vi "ep_Public Record Inf to String.vi"(8 "error in":errorcluster, 11 "task in":T1={"file refnums"=[], "Data Object"=refnum, "config info"={"station_name"="", "rec_dev_id"="", "rev_year"=1999.0, "TT"=0, "##A"=0, "##D"=0, "analog channel info"=[], "status channel info"=[], "lf"=-inf, "nrates"=65535, "samp info"=[], "initial timestamp"=timestamp(0 s since 1904-01-01), "trigger timestamp"=timestamp(0 s since 1904-01-01), "ft"=enum."Binary", "timemult"=1.0}, "public inf content"={"Source"="", "Record Type"=enum."Fault", "Phase ID"="", "Event Description"="", "Device ID"="", "Distance of Fault"=-1.0, "Distance Unit"=enum."Miles", "Max_Current"=inf, "Min_Current"=-inf, "Max_Voltage"=inf, "Min_Voltage"=-inf, "EventNoteCount"=0, "Event Information"=[]}, "private inf content"=[], "internal buffers"={"start index"=1, "config to public inf"=enum."disabled", "static config info"="", "static file_des record inf"="", "static file_des channel inf"="", "public inf"="", "private inf"=""}} {"public inf content"."Event Information"."min sample number" max=9999999999; "public inf content"."Event Information"."max sample number" max=9999999999; "config info"."nrates" max=999; "config info"."status channel info"."Dn" min=1 max=999999; "config info"."analog channel info"."An" min=1 max=999999; "config info"."trigger timestamp" format="%<%H:%M:%S%6u\n%d/%m/%Y>T"; "config info"."initial timestamp" format="%<%H:%M:%S%6u\n%d/%m/%Y>T"; "config info"."##D" max=999999; "config info"."##A" max=999999; "config info"."TT" min=1 max=999999; "config info"."rev_year" min=1999.0 max=1999.0}) -> (0 "error out":errorcluster, 2 "public record inf":string, 3 "dup task":T1={"file refnums"=[], "Data Object"=refnum, "config info"={"station_name"="", "rec_dev_id"="", "rev_year"=1999.0, "TT"=0, "##A"=0, "##D"=0, "analog channel info"=[], "status channel info"=[], "lf"=-inf, "nrates"=65535, "samp info"=[], "initial timestamp"=timestamp(0 s since 1904-01-01), "trigger timestamp"=timestamp(0 s since 1904-01-01), "ft"=enum."Binary", "timemult"=1.0}, "public inf content"={"Source"="", "Record Type"=enum."Fault", "Phase ID"="", "Event Description"="", "Device ID"="", "Distance of Fault"=-1.0, "Distance Unit"=enum."Miles", "Max_Current"=inf, "Min_Current"=-inf, "Max_Voltage"=inf, "Min_Voltage"=-inf, "EventNoteCount"=0, "Event Information"=[]}, "private inf content"=[], "internal buffers"={"start index"=1, "config to public inf"=enum."disabled", "static config info"="", "static file_des record inf"="", "static file_des channel inf"="", "public inf"="", "private inf"=""}} {"public inf content"."Event Information"."min sample number" max=9999999999; "public inf content"."Event Information"."max sample number" max=9999999999; "config info"."nrates" max=999; "config info"."status channel info"."Dn" min=1 max=999999; "config info"."analog channel info"."An" min=1 max=999999; "config info"."trigger timestamp" format="%<%H:%M:%S%6u\n%d/%m/%Y>T"; "config info"."initial timestamp" format="%<%H:%M:%S%6u\n%d/%m/%Y>T"; "config info"."##D" max=999999; "config info"."##A" max=999999; "config info"."TT" min=1 max=999999; "config info"."rev_year" min=1999.0 max=1999.0})   [LabVIEW 2014, in "NI_EP_COMTRADE.lvlib"]
uses:
  <vilib>/addons/Electrical Power/File IO/NI_EP_COMTRADE.lvlib
  <vilib>/addons/Electrical Power/File IO/COMTRADE/typedefs/ep_Task.ctl
  <vilib>/addons/Electrical Power/File IO/COMTRADE/typedefs/ep_Config Info.ctl
  <vilib>/addons/Electrical Power/File IO/COMTRADE/typedefs/ep_Analog Channel Info.ctl
  <vilib>/addons/Electrical Power/File IO/COMTRADE/typedefs/ep_Status Channel Info.ctl
  <vilib>/addons/Electrical Power/File IO/COMTRADE/typedefs/ep_File Format.ctl
  <vilib>/addons/Electrical Power/File IO/COMTRADE/typedefs/ep_Public Inf Content.ctl
  <vilib>/addons/Electrical Power/File IO/COMTRADE/typedefs/ep_Public Event Inf.ctl
  <vilib>/addons/Electrical Power/File IO/COMTRADE/typedefs/ep_Private Inf Content.ctl
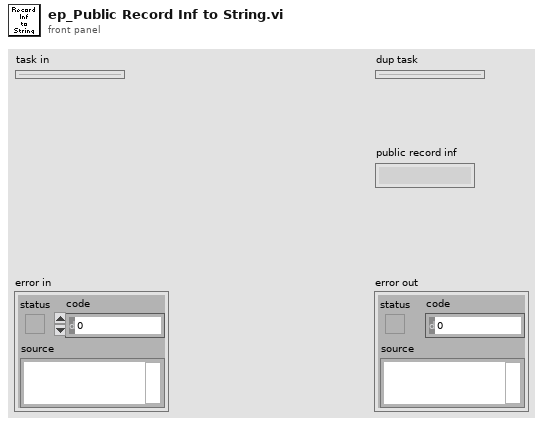
[diagram p1: front panel]
types:
  T1 = typedef "NI_EP_COMTRADE.lvlib/ep_Task.ctl" = cluster{"file refnums":refnum<file>[], "Data Object":refnum<k20>, "config info":T2, "public inf content":T6, "private inf content":T8, "internal buffers":cluster{"start index":u32, "config to public inf":enum16{"disabled", "enabled", "buffered"}, "static config info":string, "static file_des record inf":string, "static file_des channel inf":string, "public inf":string, "private inf":string}}
  T2 = typedef "NI_EP_COMTRADE.lvlib/ep_Config Info.ctl" = cluster{"station_name":string, "rec_dev_id":string, "rev_year":dbl, "TT":u32, "##A":u32, "##D":u32, "analog channel info":T3[], "status channel info":T4[], "lf":sgl, "nrates":u16, "samp info":cluster{"samp":sgl, "endsamp":u32}[], "initial timestamp":timestamp, "trigger timestamp":timestamp, "ft":T5, "timemult":sgl}
  T3 = typedef "NI_EP_COMTRADE.lvlib/ep_Analog Channel Info.ctl" = cluster{"An":u32, "ch_id":string, "ph":string, "ccbm":string, "uu":string, "a":sgl, "b":sgl, "skew":sgl, "min":i32, "max":i32, "primary":sgl, "secondary":sgl, "PS":enum16{"P", "S"}}
  T4 = typedef "NI_EP_COMTRADE.lvlib/ep_Status Channel Info.ctl" = cluster{"Dn":u32, "ch_id":string, "ph":string, "ccbm":string, "Y":bool}
  T5 = typedef "NI_EP_COMTRADE.lvlib/ep_File Format.ctl" = enum16{"ASCII", "Binary"}
  T6 = typedef "NI_EP_COMTRADE.lvlib/ep_Public Inf Content.ctl" = cluster{"Source":string, "Record Type":enum16{"Fault", "Unknown", "Misoperation", "Close", "Trip", "Reclose", "Power swing", "Simulation"}, "Phase ID":string, "Event Description":string, "Device ID":string, "Distance of Fault":dbl, "Distance Unit":enum16{"Miles", "Kilometers", "Percent of line", "Percent of setting", "Ohms"}, "Max_Current":dbl, "Min_Current":dbl, "Max_Voltage":dbl, "Min_Voltage":dbl, "EventNoteCount":u32, "Event Information":T7[]}
  T7 = typedef "NI_EP_COMTRADE.lvlib/ep_Public Event Inf.ctl" = cluster{"channel number":u32, "max value":dbl, "min value":dbl, "max sample number":u64, "min sample number":u64, "max sample text":string[], "min sample text":string[]}
  T8 = typedef "NI_EP_COMTRADE.lvlib/ep_Private Inf Content.ctl" = cluster{"Section Header":string, "Entry Names":string[], "Entry Values":string[]}[]
  T9 = enum16{"Fault", "Unknown", "Misoperation", "Close", "Trip", "Reclose", "Power Swing", "Simulation"}
  T10 = enum16{"Fault", "Unknown", "Misoperation", "Close", "Trip", "Reclose", "Power swing", "Simulation"}
  T11 = enum16{"Miles", "Kilometers", "Percent of line", "Percent of setting", "Ohms"}
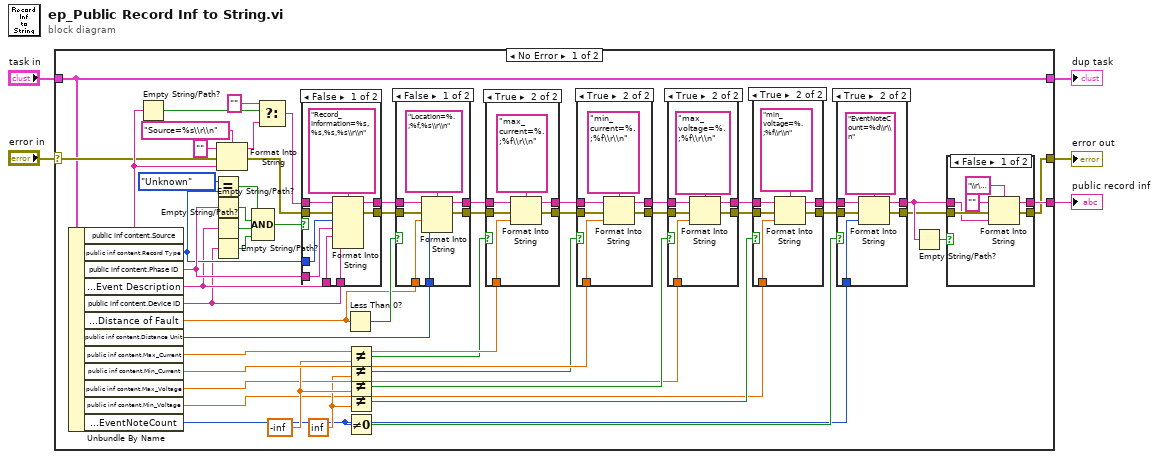
[diagram p0: block diagram]
diagram:
  n1 = case shown="No Error" "error in" {
    selector: "error in" -> [w38 w126]
    tunnel: "task in" -> [w37 w127]
    tunnel: [w37 w127] -> w3
    tunnel: [w6 w126] -> w2
    tunnel: [w9 _] -> w1
    frame No Error {
      w19 = inf ("y")
      w24 = -inf ("y")
      n2 = Unbundle By Name(w37) -> ("public inf content.Source"=w47:string, "public inf content.Record Type"=w43:T10, "public inf content.Phase ID"=w52:string, "public inf content.Event Description"=w36:string, "public inf content.Device ID"=w35:string, "public inf content.Distance of Fault"=w33:dbl, "public inf content.Distance Unit"=w34:T11, "public inf content.Max_Current"=w30:dbl, "public inf content.Min_Current"=w26:dbl, "public inf content.Max_Voltage"=w20:dbl, "public inf content.Min_Voltage"=w15:dbl, "public inf content.EventNoteCount"=w12:u32)
      n3 = Empty String/Path?(string/path=w47) -> (empty?=w49:bool)
      n4 = Equal?(x=T9."Unknown" ("y"), y=w43) -> (x = y?=w56:bool)
      n5 = Empty String/Path?(string/path=w52) -> (empty?=w55:bool)
      n6 = Empty String/Path?(string/path=w36) -> (empty?=w54:bool)
      n7 = Empty String/Path?(string/path=w35) -> (empty?=w46:bool)
      n8 = Format Into String(format string="Source=%s\\r\\n", initial string="", error in=w38, w47) -> (resulting string=w50:string, error out=w44:errorcluster)
      n9 = Compound Arithmetic op=AND(w56, w55, w54, w46) -> (w53:bool)
      n10 = Select(t="", s=w49, f=w50) -> (s? t:f=w45:string)
      n11 = case shown="False" w53 {
        tunnel: w43 -> [w123 _]
        tunnel: w52 -> [w119 _]
        tunnel: w45 -> [w121 w125]
        tunnel: w44 -> [w120 w124]
        tunnel: [w118 w124] -> w40
        tunnel: [w117 w125] -> w39
        tunnel: w36 -> [w116 _]
        tunnel: w35 -> [w115 _]
        frame False {
          n12 = Format Into String(format string="Record_Information=%s,%s,%s,%s\\r\\n", initial string=w121, error in=w120, w123, w119, w116, w115) -> (resulting string=w117:string, error out=w118:errorcluster)
        }
        frame True {
        }
      }
      n13 = Less Than 0?(x=w33) -> (x < 0?=w41:bool)
      n14 = Not Equal?(x=w30, y=w24) -> (x != y?=w27:bool)
      n15 = Not Equal?(x=w26, y=w19) -> (x != y?=w25:bool)
      n16 = Not Equal?(x=w20, y=w24) -> (x != y?=w21:bool)
      n17 = Not Equal?(x=w15, y=w19) -> (x != y?=w16:bool)
      n18 = Not Equal To 0?(x=w12) -> (x != 0?=w13:bool)
      n19 = case shown="False" w41 {
        tunnel: [w112 w114] -> w31
        tunnel: w40 -> [w109 w114]
        tunnel: [w110 w113] -> w32
        tunnel: w39 -> [w111 w113]
        tunnel: w34 -> [w108 _]
        tunnel: w33 -> [w107 _]
        frame False {
          n20 = Format Into String(format string="Location=%.;%f,%s\\r\\n", initial string=w111, error in=w109, w107, w108) -> (resulting string=w110:string, error out=w112:errorcluster)
        }
        frame True {
        }
      }
      n21 = case shown="True" w27 {
        tunnel: [w99 w105] -> w28
        tunnel: w31 -> [w99 w102]
        tunnel: [w98 w103] -> w29
        tunnel: w32 -> [w98 w104]
        tunnel: w30 -> [_ w101]
        frame False {
        }
        frame True {
          n22 = Format Into String(format string="max_current=%.;%f\\r\\n", initial string=w104, error in=w102, w101) -> (resulting string=w103:string, error out=w105:errorcluster)
        }
      }
      n23 = case shown="True" w25 {
        tunnel: [w91 w97] -> w22
        tunnel: w28 -> [w91 w94]
        tunnel: [w90 w95] -> w23
        tunnel: w29 -> [w90 w96]
        tunnel: w26 -> [_ w93]
        frame False {
        }
        frame True {
          n24 = Format Into String(format string="min_current=%.;%f\\r\\n", initial string=w96, error in=w94, w93) -> (resulting string=w95:string, error out=w97:errorcluster)
        }
      }
      n25 = case shown="True" w21 {
        tunnel: [w83 w89] -> w17
        tunnel: w22 -> [w83 w86]
        tunnel: [w82 w87] -> w18
        tunnel: w23 -> [w82 w88]
        tunnel: w20 -> [_ w85]
        frame False {
        }
        frame True {
          n26 = Format Into String(format string="max_voltage=%.;%f\\r\\n", initial string=w88, error in=w86, w85) -> (resulting string=w87:string, error out=w89:errorcluster)
        }
      }
      n27 = case shown="True" w16 {
        tunnel: [w75 w81] -> w11
        tunnel: w17 -> [w75 w78]
        tunnel: [w74 w79] -> w14
        tunnel: w18 -> [w74 w80]
        tunnel: w15 -> [_ w77]
        frame False {
        }
        frame True {
          n28 = Format Into String(format string="min_voltage=%.;%f\\r\\n", initial string=w80, error in=w78, w77) -> (resulting string=w79:string, error out=w81:errorcluster)
        }
      }
      n29 = case shown="True" w13 {
        tunnel: [w67 w73] -> w7
        tunnel: w11 -> [w67 w70]
        tunnel: [w66 w71] -> w8
        tunnel: w14 -> [w66 w72]
        tunnel: w12 -> [_ w68]
        frame False {
        }
        frame True {
          n30 = Format Into String(format string="EventNoteCount=%d\\r\\n", initial string=w72, error in=w70, w68) -> (resulting string=w71:string, error out=w73:errorcluster)
        }
      }
      n31 = Empty String/Path?(string/path=w8) -> (empty?=w10:bool)
      n32 = case shown="False" w10 {
        tunnel: [w61 w64] -> w6
        tunnel: w7 -> [w63 w64]
        tunnel: [w62 w65] -> w9
        tunnel: w8 -> [w60 w65]
        frame False {
          n33 = Format Into String(format string="\\r\\n[Public Record_Information]\\r\\n%s", initial string="", error in=w63, w60) -> (resulting string=w62:string, error out=w61:errorcluster)
        }
        frame True {
        }
      }
    }
    frame Error {
    }
  }
  "public record inf" <- w1
  "dup task" <- w3
  "error out" <- w2
